vi "NI VeriStand - Start Single Waveform (DBL).vi"(8 "error in (no error)":errorcluster, 10 "t0":timestamp, 11 "Single Waveform Write Session (DBL) in":refnum<class "Single Waveform Write (DBL).lvclass">) -> (0 "error out":errorcluster, 3 "Single Waveform Write Session (DBL) out":refnum<class "Single Waveform Write (DBL).lvclass">)   [LabVIEW 2020, in "NI_VS Custom Device Waveform API.lvlib" / "Single Waveform Write (DBL).lvclass"]
doc: "Sets the start time (t0) for the waveform data you want to write with the Write Waveform(s) VI. NI VeriStand considers all data the custom device writes to a waveform be continuous unless this VI executes again with a different start time."
uses:
  Single Waveform Write (DBL).lvclass
  D:/p4/penguin/lvaddon/Veristand/master/src/LabVIEW/vilib/NI VeriStand/Custom Device Waveform API/Waveform Session.lvclass
  Waveform Session.lvclass/Waveform Session.ctl
  Single Waveform Write (DBL).lvclass/Single Waveform Write (DBL).ctl
  Internal Comm Classes/WPL Comm/WPL Comm.lvclass/WPL Comm.ctl
  Internal Comm Classes/WPL Comm/Set t0 on Variant.vi
  Internal Comm Classes/WPL Comm/Send WPL Command.vi
  Internal Comm Classes/WPL Comm/Convert Q Error to Shutdown Error.vi
  Internal Comm Classes/WPL Comm/WPL Comm (1D DBL)/WPL Comm (1D DBL).lvclass
  D:/p4/penguin/lvaddon/Veristand/master/src/LabVIEW/vilib/NI VeriStand/Custom Device Waveform API/Internal Comm Classes/WPL Comm/WPL Comm.lvclass
  <vilib>/Utility/error.llb/Error Cluster From Error Code.vi
  Internal Comm Classes/WPL Comm/WPL Comm.lvclass
  Waveform Session.lvclass
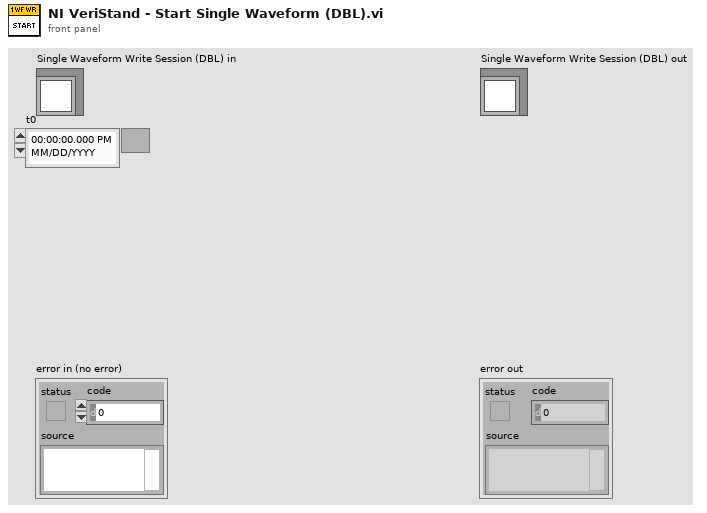
[diagram p1: front panel]
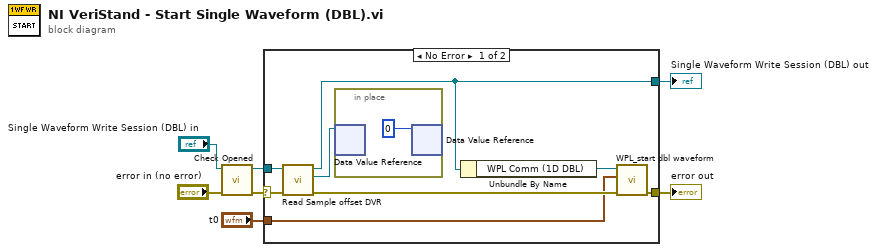
[diagram p0: block diagram]
diagram:
  n1 = call "Check Opened.vi"("error in (no error)"="error in (no error)", "Waveform Session in"="Single Waveform Write Session (DBL) in") -> ("error out"=w2:errorcluster, "Waveform Session out"=w1:refnum<class "Single Waveform Write (DBL).lvclass">)  [unwired: 8 in]
  n2 = case shown="No Error" w2 {
    selector: w2 -> [w14 w17]
    tunnel: [w12 w17] -> w7
    tunnel: [w8 w16] -> w6
    tunnel: w1 -> [w10 w16]
    tunnel: "t0" -> [w11 _]
    frame No Error {
      n3 = call "Read Sample offset DVR.vi"("Waveform Session in"=w10) -> ("Sample offset"=w9:refnum<data-value>, "Waveform Session out"=w8:refnum<class "Single Waveform Write (DBL).lvclass">)  [unwired: 9 in]
      n4 = in-place {
        n5 = in-place-dvr #1(w9) -> ()  [unwired: 2 out]
        n6 = in-place-dvr #1(u64 0 ("data value")) -> ()  [unwired: 2 out]
      }
      n7 = Unbundle By Name(w8) -> ("WPL Comm (1D DBL)"=w13:refnum<class "WPL Comm (1D DBL).lvclass">)
      n8 = call "WPL_start dbl waveform.vi"("error in (no error)"=w14, "t0"=w11, "WPL Comm in"=w13) -> ("error out"=w12:errorcluster)  [unwired: 8 in]
    }
    frame Error {
    }
  }
  "error out" <- w7
  "Single Waveform Write Session (DBL) out" <- w6
